vi "PI_GCS2_Sample_Application_DataRecorder.vi"() -> ()   [LabVIEW 2020]
doc: "This VI demonstrates how to use the PI GCS3 data recorder functionality. The diagram shows how to combine the driver VIs for these tasks.\n\nWarning: Before running this VI, modify the interface settings on the block diagram to reflect your configuration. The predefined settings provided with the VI probably do not match your system.\n\nCompatibility: This sample requires a PI GCS 3.0 controller."
uses:
  Low Level/Communication/Interface Settings.ctl
panel:
  out "Recorded data points":i32[](array[numeric])
  out "Position Error of AXIS_1":waveform(dbl)(graph)
  out "Generated Position of AXIS_1":waveform(dbl)(graph)
  out "Real Position of AXIS_1":waveform(dbl)(graph)
  out "Conn. Axes":string[](array[string])
  out "Identification":string
  out "error out":errorcluster
  in  "error in (no error)":errorcluster
  # "This VI demonstrates how to use the PI GCS2 data recorder functionality.\nThe diagram shows how to combine the driver VIs for these tasks. \n\nWarning: Before running this VI, modify the interface settings on the block diagram to reflect your configuration.\n                 The predefined settings provided with the VI probably do not match your system.\n\nCompatibility: This sample requires a PI GCS 2.0 controller."
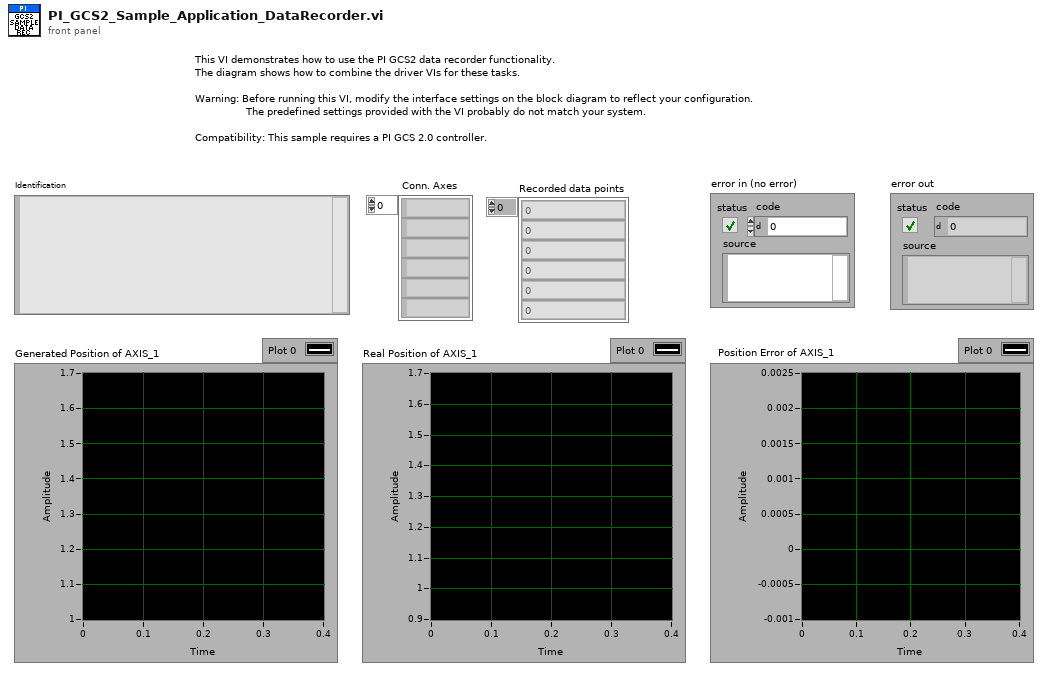
[diagram p1: front panel]
types:
  T1 = enum16{"Do not reference", "Reference switch", "Negative limit switch", "Positive limit switch"}[]
  T2 = typedef "Interface Settings.ctl" = cluster{"Interface":u16, "Timeout":u32, "RS232 settings":cluster{"Portnumber":u8, "Baudrate":u16}, "TCP/IP settings":cluster{"Host address/name":string, "Port":i32, "Board":i32, "TCP/IP Search?":bool}, "USB settings":cluster{"S/N":string, "USB Search?":bool}, "DaisyChain settings":cluster{"Register DC":bool, "DaisyChain Search?":bool, "Device ID":i32}, "DLL for Device":u16}
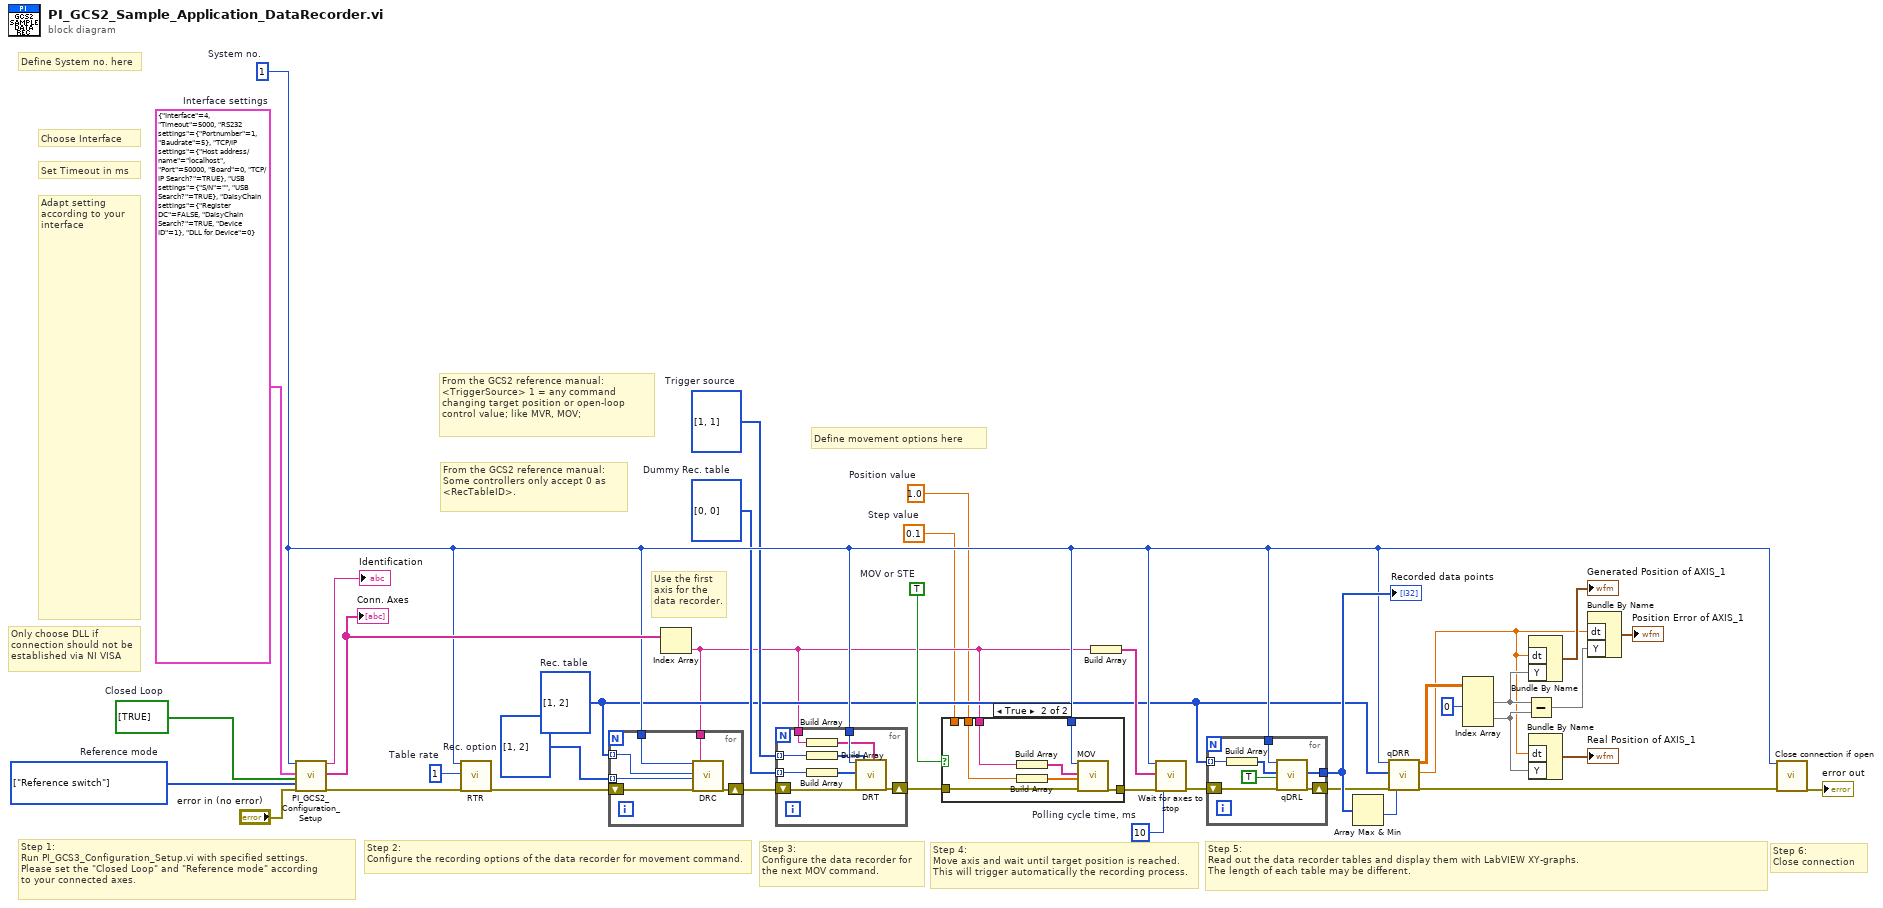
[diagram p0: block diagram]
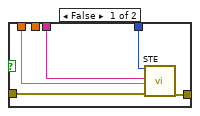
[diagram p2: hidden frame]
diagram:
  w2 = 0.1  # Step value
  w1 = 1.0  # Position value
  w13 = TRUE  # MOV or STE
  w6 = i32[] [0, 0]  # Dummy Rec. table
  w15 = u32 10  # Polling cycle time, ms
  w24 = i32[] [1, 2]  # Rec. option
  w4 = i32[] [1, 2]  # Rec. table
  w5 = i32[] [1, 1]  # Trigger source
  w25 = 1  # Table rate
  w26 = T1 [enum."Reference switch"] items=["Do not reference", "Reference switch", "Negative limit switch", "Positive limit switch"]  # Reference mode
  w27 = bool[] [TRUE]  # Closed Loop
  w28 = T2 {"Interface"=4, "Timeout"=5000, "RS232 settings"={"Portnumber"=1, "Baudrate"=5}, "TCP/IP settings"={"Host address/name"="localhost", "Port"=50000, "Board"=0, "TCP/IP Search?"=TRUE}, "USB settings"={"S/N"="", "USB Search?"=TRUE}, "DaisyChain settings"={"Register DC"=FALSE, "DaisyChain Search?"=TRUE, "Device ID"=1}, "DLL for Device"=0}  # Interface settings
  w7 = 1  # System no.
  # "Use the first\naxis for the\ndata recorder."
  # "Define movement options here"
  # "From the GCS2 reference manual:\nSome controllers only accept 0 as <RecTableID>."
  # "From the GCS2 reference manual:\n<TriggerSource> 1 = any command changing target position or open-loop control value; like MVR, MOV;"
  # "Define System no. here"
  # "Adapt setting according to your interface"
  # "Set Timeout in ms"
  # "Choose Interface"
  # "Only choose DLL if connection should not be established via NI VISA"
  # "Step 4:\nMove axis and wait until target position is reached. This will trigger automatically the recording process."
  # "Step 5:\nRead out the data recorder tables and display them with LabVIEW XY-graphs.\nThe length of each table may be different."
  # "Step 3:\nConfigure the data recorder for the next MOV command."
  # "Step 2:\nConfigure the recording options of the data recorder for movement command."
  # "Step 6:\nClose connection"
  # "Step 1:\nRun PI_GCS3_Configuration_Setup.vi with specified settings.\nPlease set the \"Closed Loop\" and \"Reference mode\" according\nto your connected axes."
  n1 = call "PI_GCS2_Configuration_Setup.vi"("System no."=w7, "Interface settings"=w28, "Closed Loop"=w27, "Reference mode"=w26, "error in"="error in (no error)") -> ("Identification"=→"Identification":string, "Conn. Axis"=w16:string[], "error out"=w21:errorcluster)  [unwired: 9 in, 3 out]
  "Conn. Axes" <- w16
  n2 = call "RTR.vi"("System no."=w7, "Table rate"=w25, "error in"=w21) -> ("error out"=w23:errorcluster)  [unwired: 15 in, 1 out]
  n3 = Index Array(array=w16) -> (element=w3:string)  [unwired: 1 in]
  n4 = for {
    tunnel: w4 -> [w44] mode=indexing
    tunnel: w24 -> [w43] mode=indexing
    shift-right: [w42] -> w9
    shift-left: w23 -> [w41]
    tunnel: w7 -> [w40]
    tunnel: w3 -> [w39]
    n5 = call "DRC.vi"("System no."=w40, "Rec. table"=w44, "Rec. option"=w43, "error in"=w41, "Source ID"=w39) -> ("error out"=w42:errorcluster)  [unwired: 13 in, 1 out]
  }
  n6 = for {
    shift-right: [w52] -> w8
    shift-left: w9 -> [w53]
    tunnel: w7 -> [w51]
    tunnel: w3 -> [w49]
    tunnel: w6 -> [w48] mode=indexing
    tunnel: w5 -> [w46] mode=indexing
    n7 = Build Array(w49) -> (w50:string[])
    n8 = Build Array(w46) -> (w45:i32[])
    n9 = Build Array(w48) -> (w47:i32[])
    n10 = call "DRT.vi"("System no."=w51, "DataRecorderTable"=w47, "error in"=w53, "Trigger source"=w45, "Value"=w50) -> ("error out"=w52:errorcluster)  [unwired: 13 in, 1 out]
  }
  n11 = case shown="True" w13 {
    tunnel: [w58 w65] -> w38
    tunnel: w8 -> [w57 w64]
    tunnel: w7 -> [w56 w63]
    tunnel: w3 -> [w55 w62]
    tunnel: w2 -> [w54 _]
    tunnel: w1 -> [_ w59]
    frame False {
      n12 = call "STE.vi"("System no."=w56, "Axis to command"=w55, "Step size"=w54, "error in"=w57) -> ("error out"=w58:errorcluster)  [unwired: 15 in]
    }
    frame True {
      n13 = Build Array(w62) -> (w61:string[])
      n14 = Build Array(w59) -> (w60:dbl[])
      n15 = call "MOV.vi"("System no."=w63, "Axes to move"=w61, "Position values"=w60, "error in"=w64) -> ("error out"=w65:errorcluster)  [unwired: 15 in]
    }
  }
  n16 = Build Array(w3) -> (w11:string[])
  n17 = call "Wait for axes to stop.vi"("System no."=w7, "Axes to wait for"=w11, "error in"=w38, "Polling cycle time, ms"=w15) -> ("error out"=w12:errorcluster)  [unwired: 14 in, 1 out]
  n18 = for {
    tunnel: [w71] -> w17
    tunnel: w7 -> [w68]
    shift-right: [w69] -> w10
    shift-left: w12 -> [w70]
    tunnel: w4 -> [w66] mode=indexing
    n19 = Build Array(w66) -> (w67:i32[])
    n20 = call "qDRL.vi"("System no."=w68, "Rec. table to query"=w67, "With Rec. table IDs?"=TRUE, "error in"=w70) -> ("No. of rec. values"=w71:i32[], "error out"=w69:errorcluster)  [unwired: 14 in]
  }
  "Recorded data points" <- w17
  n21 = Array Max & Min(array=w17) -> (min value=w22:i32)  [unwired: 3 out]
  n22 = call "qDRR.vi"("System no."=w7, "Rec. table IDs"=w4, "error in"=w10, "N"=w22) -> ("Data"=w19:dbl[][], "Sample Time"=w18:dbl, "error out"=w20:errorcluster)  [unwired: 11 in, 2 out]
  n23 = Index Array(array=w19, index (col) #1=0 ("disabled index (col)")) -> (element #1=w34:dbl[], element #2=w33:dbl[])  [unwired: 3 in]
  n24 = Subtract(x=w34, y=w33) -> (x-y=w32:dbl[])
  n25 = Bundle By Name("dt"=w18, "Y"=w34) -> (→"Generated Position of AXIS_1":waveform(dbl))  [unwired: 1 in]
  n26 = Bundle By Name("dt"=w18, "Y"=w33) -> (→"Real Position of AXIS_1":waveform(dbl))  [unwired: 1 in]
  n27 = Bundle By Name("dt"=w18, "Y"=w32) -> (→"Position Error of AXIS_1":waveform(dbl))  [unwired: 1 in]
  n28 = call "Close connection if open.vi"("System no."=w7, "error in"=w20) -> ("error out"=→"error out":errorcluster)  [unwired: 16 in, 1 out]
